vi "Device Deactivate.vi"(8 "error in (no error)":errorcluster, 10 "Activate Mode":T1, 11 "IED in":refnum<class "IED.lvclass">) -> (0 "error out":errorcluster, 3 "IED out":refnum<class "IED.lvclass">)   [LabVIEW 2015, in "IED Actor.lvlib" / "IED.lvclass"]
uses:
  IED.lvclass
  Controls/Device Deactivate Mode Select.ctl
  <vilib>/ActorFramework/Actor/Actor.lvclass/Actor.ctl
  IED.lvclass/IED.ctl
  SCADA Core/SCADA Abstract Messages/Simple Command Status Msg/Simple Command Status.ctl
  SCADA Core/SCADA Response Messages/Return Shutdown Status Msg/Return Shutdown Status Msg.lvclass/Return Shutdown Status Msg.ctl
  <vilib>/ActorFramework/Message Enqueuer/Message Enqueuer.lvclass/Message Enqueuer.ctl
  SCADA Core/SCADA Messages/Return Island Status Msg/Return Island Status Msg.lvclass/Return Island Status Msg.ctl
  <vilib>/ActorFramework/Message Enqueuer/Enqueue.vi
  <vilib>/ActorFramework/Message Priority Queue/Priority Enqueue.vi
  SCADA Core/SCADA Response Messages/Return Shutdown Status Msg/Return Shutdown Status Msg.lvclass
  SCADA Core/SCADA Messages/Return Island Status Msg/Return Island Status Msg.lvclass
  <vilib>/Modbus/master/Modbus Master.lvclass
  <vilib>/ActorFramework/Actor/Actor.lvclass
  SCADA Core/SCADA Abstract Messages/Simple Command Status Msg/Simple Command Status Msg.lvclass
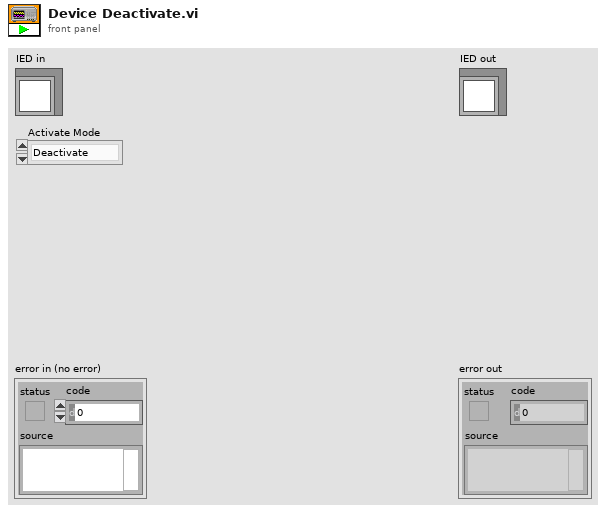
[diagram p1: front panel]
types:
  T1 = typedef "IED Actor.lvlib/IED.lvclass/Device Deactivate Mode Select.ctl" = enum16{"Deactivate", "Shutdown", "Island"}
  T2 = typedef "SCADA Core.lvlib/Simple Command Status Msg.lvclass/Simple Command Status.ctl" = enum16{"Success", "Failure"}
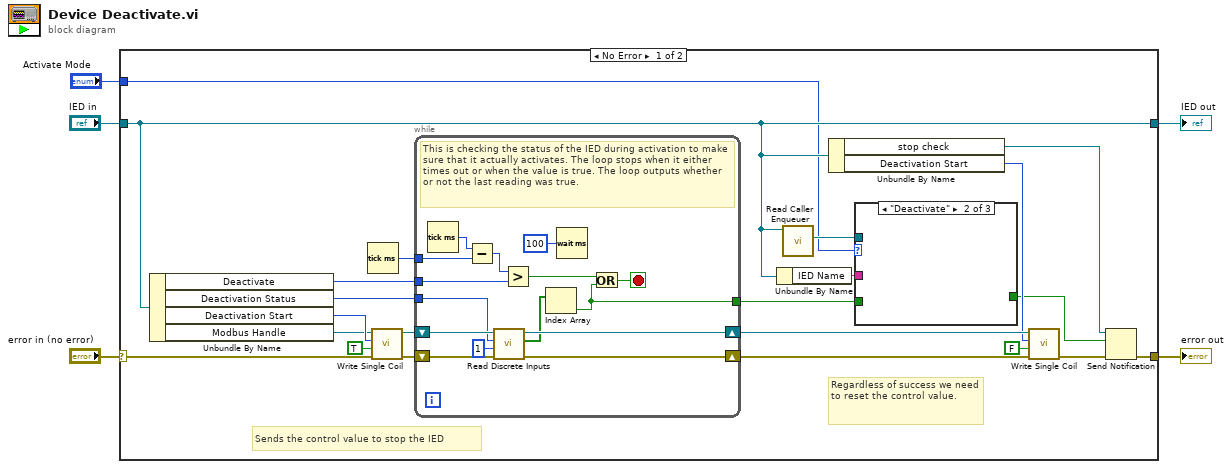
[diagram p0: block diagram]
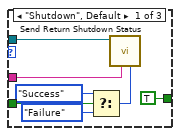
[diagram p2: hidden frame]
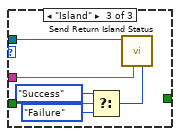
[diagram p3: hidden frame]
diagram:
  n1 = case shown="No Error" "error in (no error)" {
    selector: "error in (no error)" -> [w9 w57]
    tunnel: [w14 w57] -> w4
    tunnel: [w11 w56] -> w2
    tunnel: "IED in" -> [w11 w56]
    tunnel: "Activate Mode" -> [w10 _]
    frame No Error {
      # "Regardless of success we need to reset the control value."
      # "Sends the control value to stop the IED"
      n2 = Unbundle By Name(w11) -> ("Deactivate"=w21:u32, "Deactivation Status"=w22:u16, "Deactivation Start"=w26:u16, "Modbus Handle"=w8:refnum<class "Modbus Master.lvclass">)
      n3 = Tick Count (ms)() -> (millisecond timer value=w27:u32)
      n4 = call-dynamic "Write Single Coil.vi"("error in (no error)"=w9, "coil value"=TRUE, "address"=w26, "Modbus master in"=w8) -> ("error out"=w23:errorcluster, "Modbus master out"=w24:refnum<class "Modbus Master.lvclass">)  [unwired: 6 in]
      n5 = while {
        tunnel: w27 -> [w53]
        tunnel: w21 -> [w51]
        tunnel: w22 -> [w47]
        shift-right: [w41] -> w20
        shift-left: w23 -> [w46]
        tunnel: [w42] -> w15
        shift-right: [w44] -> w19
        shift-left: w24 -> [w48]
        stop <- w49 stop-if-true
        # "This is checking the status of the IED during activation to make sure that it actually activates. The loop stops when it either times out or when the value is true. The loop outputs whether or not the last reading was true."
        n6 = Tick Count (ms)() -> (millisecond timer value=w54:u32)
        n7 = Subtract(x=w54, y=w53) -> (x-y=w52:u32)
        n8 = call-dynamic "Read Discrete Inputs.vi"("error in (no error)"=w46, "number of discrete inputs"=u16 1 ("number of coils"), "starting address"=w47, "Modbus master in"=w48) -> ("error out"=w41:errorcluster, "discrete input values"=w43:bool[], "Modbus master out"=w44:refnum<class "Modbus Master.lvclass">)  [unwired: 5 in]
        n9 = Greater?(x=w52, y=w51) -> (0:w50:bool)
        n10 = Index Array(array=w43) -> (element=w42:bool)  [unwired: 1 in]
        n11 = Wait (ms)(milliseconds to wait=u32 100) -> ()  [unwired: 1 out]
        n12 = Or(x=w50, y=w42) -> (x .or. y?=w49:bool)
      }
      n13 = Unbundle By Name(w11) -> ("IED Name"=w12:string)
      n14 = call <vilib>:"Read Caller Enqueuer.vi"("Actor"=w11) -> ("Caller Enqueuer"=w16:refnum<class "Message Enqueuer.lvclass">)  [unwired: 10 in]
      n15 = Unbundle By Name(w11) -> ("stop check"=w13:refnum<notifier>, "Deactivation Start"=w18:u16)
      n16 = case shown="\"Deactivate\"" w10 {
        tunnel: w16 -> [w34 _ w37]
        tunnel: w15 -> [w33 _ w40]
        tunnel: w12 -> [w29 _ w36]
        tunnel: [TRUE ("notification") _ _] -> w6
        frame "Shutdown", Default {
          n17 = Select(t=Simple_Command_Status."Success" ("Status"), s=w33, f=Simple_Command_Status."Failure" ("Status")) -> (s? t:f=w30:T2)
          n18 = call "Send Return Shutdown Status.vi"("Status"=w30, "error"=w29, "Message Enqueuer"=w34) -> ()  [unwired: 7 in, 2 out]
        }
        frame "Deactivate" {
        }
        frame "Island" {
          n19 = Select(t=Simple_Command_Status."Success" ("Status"), s=w40, f=Simple_Command_Status."Failure" ("Status")) -> (s? t:f=w35:T2)
          n20 = call "Send Return Island Status.vi"("Status"=w35, "error"=w36, "Message Enqueuer"=w37) -> ()  [unwired: 7 in, 2 out]
        }
      }
      n21 = call-dynamic "Write Single Coil.vi"("error in (no error)"=w20, "coil value"=FALSE, "address"=w18, "Modbus master in"=w19) -> ("error out"=w7:errorcluster)  [unwired: 6 in, 1 out]
      n22 = Send Notification(notification=w6, notifier=w13, error in (no error)=w7) -> (error out=w14:errorcluster)  [unwired: 1 out]
    }
    frame Error {
    }
  }
  "error out" <- w4
  "IED out" <- w2
